vi "ExpStateLoadBridge.vi"(8 "Error In":errorcluster, 11 "Experiment State IN":T17={"error"={"status"=FALSE, "code"=0, "source"=""}, "Digitizer DAQmx Tasks"={"TaskArray"=[]}, "DAQ Settings"={"Channel Settings"=[], "Card Settings"=[]}, "Synchronization Settings"={"Synchronizer 0"="PXI1Slot2", "source terminal"="GlobalSoftwareTrigger", "Synchronizer 1"="PXI1Slot2"}, "DAQ Data"=[], "Next Shot#"="0", "System Message"="", "User Shot Notes"="", "Timing Settings"={"Timing Card Settings"=[], "Timing Channel Settings"=[[{"Delay (s)"=2.559999942779541, "Pulse width (s)"=0.009999999776482582, "Active"=TRUE, "Channel Name"="Fiber 8", "counter"="PXI1Slot8/ctr7", "FrontPanelTime"=2.559999942779541}]]}, "Timing Tasks"={"TaskArray"=[]}, "Tree"="0", "Time Card/Channels"=[2, 8], "DAQ Card/Channels"=[3, 8], "Program Version"="", "RIO Settings"={"Channel Settings"=[], "Card Settings"=[]}, "RIO References"={"Reference Array"=[]}, "RIO Data"={"RIO Deleaved Data"=[], "Raw Readout"=[]}, "RIO Card/Channels"=[3, 8], "DIO Channels"=0, "DIO Settings"={"DIO Channel Array"=[]}, "Global Settings"={"Initial Background Values"={"Reference Shot #"=0.0, "Background pressure [Torr]"=0.0, "Cryo temp [V]"=0.0, "Cryo temp [K]"=0.0, "Cryotemp Calibration File"=path ""}, "Gas Puffing"={"Gas A type"="N", "Gas B type"="N", "Gas C type"="N", "Gas A pressure [psi]"=0.0, "Gas B pressure [psi]"=0.0, "Gas C pressure [psi]"=0.0, "Innner Electrode"="", "Middle Electrode"="", "Outer Electrode"="", "Gas A bottle pressure [psi]"=0.0, "Gas B bottle pressure [psi]"=0.0, "Gas C bottle pressure [psi]"=0.0}, "PSU Voltages"={"Bias1 Voltage [V]"=0.0, "Bias2 Voltage [V]"=0.0, "PSU1 Voltage [V]"=0.0, "Puff-PSU1 CH1 Voltage [V]"=0.0, "Puff-PSU1 CH2 Voltage [V]"=0.0, "Puff-PSU1 CH3 Voltage [V]"=0.0, "PSU2 Voltage [V]"=0.0, "PSU3 Voltage [V]"=0.0}, "TEK 2024B - TEK - Details"={"CH1"="", "CH2"="", "CH3"="", "CH4"="", "CH1 Ground State"="Grounded", "CH2 Ground State"="Grounded", "CH3 Ground State"="Grounded", "CH4 Ground State"="Grounded"}, "TEK 2024B - TEK1 - Details"={"CH1"="", "CH2"="", "CH3"="", "CH4"="", "CH1 Ground State"="Grounded", "CH2 Ground State"="Grounded", "CH3 Ground State"="Grounded", "CH4 Ground State"="Grounded"}}, "Calibrations"={"CryoTemp"={"Comment"="", "X"=[], "Y"=[]}, "PSU2 Tach"={"Comment"="", "X"=[], "Y"=[]}, "PSU3 Tach"={"Comment"="", "X"=[], "Y"=[]}, "PSU2 RevTach"={"Comment"="", "X"=[], "Y"=[]}, "PSU3 RevTach"={"Comment"="", "X"=[], "Y"=[]}}, "Tach Tasks"={"PSU2 task"="", "PSU3 task"=""}, "PSU2 Panel Settings"={"PSU2 DIO channels"={"Charge relay DIO"="DAQ0/port0/line3", "Dump relay DIO"="DAQ0/port0/line4", "HV Arm DIO"="DAQ0/port0/line5", "HV On DIO"="DAQ0/port0/line6"}, "PSU2 Tachometer Controls"={"PSU2 Tach Calibration"=path "Z:/Data/Calibration/Tachometer", "PSU2 Charging Voltage [kV]"=0.0, "PSU2 Tach Counter"="DAQ0/port0/line3"}, "PSU2 Reverse Tachometer Controls"={"PSU2 RevTach Calibration"=path "Z:/Data/Calibration/Reverse Tachometer/PSU2_RevTachCalibration.csv", "PSU2 bank Voltage [kV]"=0.0, "PSU2 RevTach Counter"=""}}, "PSU3 Panel Settings"={"PSU3 DIO channels"={"Charge relay DIO"="DAQ0/port0/line5", "Dump relay DIO"="DAQ0/port0/line6", "HV Arm DIO"="", "HV On DIO"="DAQ0/port0/line6"}, "PSU3 Tachometer Controls"={"PSU3 Tach Calibration"=path "Z:/Data/Calibration/Reverse Tachometer/PSU3_RevTachCalibration.csv", "PSU3 Charging Voltage [kV]"=0.0, "PSU3 Tach Counter"=""}, "PSU3 Reverse Tachometer Controls"={"PSU3 RevTach Calibration"=path "Z:/Data/Calibration/Reverse Tachometer/PSU3_RevTachCalibration.csv", "PSU3 bank Voltage [kV]"=0.0, "PSU3 RevTach Counter"=""}}} {"Global Settings"."Initial Background Values"."Cryo temp [K]" format="%#_4g"; "RIO Settings"."Card Settings"."Digital High \nPass Filter k" items=["10"=21, "9"=19, "8"=17, "7"=15, "6"=13, "5"=11, "4"=9, "3"=7, "2"=5, "Off"=0]; "RIO Settings"."Card Settings"."Sample Rate" format="%#_3p"; "Timing Settings"."Timing Channel Settings"."FrontPanelTime" format="%.3p"; "Timing Settings"."Timing Channel Settings"."Pulse width (s)" format="%.3p"; "Timing Settings"."Timing Channel Settings"."Delay (s)" format="%.3p"; "DAQ Settings"."Card Settings"."Global Edge Type" items=["Rising"=10280, "Falling"=10171]; "DAQ Settings"."Card Settings"."Sample Rate" format="%#_3p"}) -> (0 "Load RIO Array":T7 {"Card Settings"."Digital High \nPass Filter k" items=["10"=21, "9"=19, "8"=17, "7"=15, "6"=13, "5"=11, "4"=9, "3"=7, "2"=5, "Off"=0]; "Card Settings"."Start Time" format="%#_3p"; "Card Settings"."End Time" format="%#_3p"; "Card Settings"."Rate" format="%#_3p"}, 1 "Load DAQ Array":T46(array[cluster]) {"Card Settings"."Start Time" format="%#_3p"; "Card Settings"."End Time" format="%#_3p"; "Card Settings"."Rate" format="%#_3p"}, 2 "Load Timing Array":T47[](array[typedef]) {"Timing Sequence"."Pulse Width [s]" format="%#.2p"; "Timing Sequence"."Dt" format="%.2p"; "Timing Sequence"."Time" format="%.2p"}, 3 "Experiment State OUT":T17={"error"={"status"=FALSE, "code"=0, "source"=""}, "Digitizer DAQmx Tasks"={"TaskArray"=[]}, "DAQ Settings"={"Channel Settings"=[], "Card Settings"=[]}, "Synchronization Settings"={"Synchronizer 0"="PXI1Slot2", "source terminal"="GlobalSoftwareTrigger", "Synchronizer 1"="PXI1Slot2"}, "DAQ Data"=[], "Next Shot#"="0", "System Message"="", "User Shot Notes"="", "Timing Settings"={"Timing Card Settings"=[], "Timing Channel Settings"=[[{"Delay (s)"=2.559999942779541, "Pulse width (s)"=0.009999999776482582, "Active"=TRUE, "Channel Name"="Fiber 8", "counter"="PXI1Slot8/ctr7", "FrontPanelTime"=2.559999942779541}]]}, "Timing Tasks"={"TaskArray"=[]}, "Tree"="0", "Time Card/Channels"=[2, 8], "DAQ Card/Channels"=[3, 8], "Program Version"="", "RIO Settings"={"Channel Settings"=[], "Card Settings"=[]}, "RIO References"={"Reference Array"=[]}, "RIO Data"={"RIO Deleaved Data"=[], "Raw Readout"=[]}, "RIO Card/Channels"=[3, 8], "DIO Channels"=0, "DIO Settings"={"DIO Channel Array"=[]}, "Global Settings"={"Initial Background Values"={"Reference Shot #"=0.0, "Background pressure [Torr]"=0.0, "Cryo temp [V]"=0.0, "Cryo temp [K]"=0.0, "Cryotemp Calibration File"=path ""}, "Gas Puffing"={"Gas A type"="N", "Gas B type"="N", "Gas C type"="N", "Gas A pressure [psi]"=0.0, "Gas B pressure [psi]"=0.0, "Gas C pressure [psi]"=0.0, "Innner Electrode"="", "Middle Electrode"="", "Outer Electrode"="", "Gas A bottle pressure [psi]"=0.0, "Gas B bottle pressure [psi]"=0.0, "Gas C bottle pressure [psi]"=0.0}, "PSU Voltages"={"Bias1 Voltage [V]"=0.0, "Bias2 Voltage [V]"=0.0, "PSU1 Voltage [V]"=0.0, "Puff-PSU1 CH1 Voltage [V]"=0.0, "Puff-PSU1 CH2 Voltage [V]"=0.0, "Puff-PSU1 CH3 Voltage [V]"=0.0, "PSU2 Voltage [V]"=0.0, "PSU3 Voltage [V]"=0.0}, "TEK 2024B - TEK - Details"={"CH1"="", "CH2"="", "CH3"="", "CH4"="", "CH1 Ground State"="Grounded", "CH2 Ground State"="Grounded", "CH3 Ground State"="Grounded", "CH4 Ground State"="Grounded"}, "TEK 2024B - TEK1 - Details"={"CH1"="", "CH2"="", "CH3"="", "CH4"="", "CH1 Ground State"="Grounded", "CH2 Ground State"="Grounded", "CH3 Ground State"="Grounded", "CH4 Ground State"="Grounded"}}, "Calibrations"={"CryoTemp"={"Comment"="", "X"=[], "Y"=[]}, "PSU2 Tach"={"Comment"="", "X"=[], "Y"=[]}, "PSU3 Tach"={"Comment"="", "X"=[], "Y"=[]}, "PSU2 RevTach"={"Comment"="", "X"=[], "Y"=[]}, "PSU3 RevTach"={"Comment"="", "X"=[], "Y"=[]}}, "Tach Tasks"={"PSU2 task"="", "PSU3 task"=""}, "PSU2 Panel Settings"={"PSU2 DIO channels"={"Charge relay DIO"="DAQ0/port0/line3", "Dump relay DIO"="DAQ0/port0/line4", "HV Arm DIO"="DAQ0/port0/line5", "HV On DIO"="DAQ0/port0/line6"}, "PSU2 Tachometer Controls"={"PSU2 Tach Calibration"=path "Z:/Data/Calibration/Tachometer", "PSU2 Charging Voltage [kV]"=0.0, "PSU2 Tach Counter"="DAQ0/port0/line3"}, "PSU2 Reverse Tachometer Controls"={"PSU2 RevTach Calibration"=path "Z:/Data/Calibration/Reverse Tachometer/PSU2_RevTachCalibration.csv", "PSU2 bank Voltage [kV]"=0.0, "PSU2 RevTach Counter"=""}}, "PSU3 Panel Settings"={"PSU3 DIO channels"={"Charge relay DIO"="DAQ0/port0/line5", "Dump relay DIO"="DAQ0/port0/line6", "HV Arm DIO"="", "HV On DIO"="DAQ0/port0/line6"}, "PSU3 Tachometer Controls"={"PSU3 Tach Calibration"=path "Z:/Data/Calibration/Reverse Tachometer/PSU3_RevTachCalibration.csv", "PSU3 Charging Voltage [kV]"=0.0, "PSU3 Tach Counter"=""}, "PSU3 Reverse Tachometer Controls"={"PSU3 RevTach Calibration"=path "Z:/Data/Calibration/Reverse Tachometer/PSU3_RevTachCalibration.csv", "PSU3 bank Voltage [kV]"=0.0, "PSU3 RevTach Counter"=""}}} {"Global Settings"."Initial Background Values"."Cryo temp [K]" format="%#_4g"; "RIO Settings"."Card Settings"."Digital High \nPass Filter k" items=["10"=21, "9"=19, "8"=17, "7"=15, "6"=13, "5"=11, "4"=9, "3"=7, "2"=5, "Off"=0]; "RIO Settings"."Card Settings"."Sample Rate" format="%#_3p"; "Timing Settings"."Timing Channel Settings"."FrontPanelTime" format="%.3p"; "Timing Settings"."Timing Channel Settings"."Pulse width (s)" format="%.3p"; "Timing Settings"."Timing Channel Settings"."Delay (s)" format="%.3p"; "DAQ Settings"."Card Settings"."Global Edge Type" items=["Rising"=10280, "Falling"=10171]; "DAQ Settings"."Card Settings"."Sample Rate" format="%#_3p"}, 4 "Load DIO Cluster":T14, 5 "Shot Notes":string, 6 "Global Settings":T2={"Initial Background Values"={"Reference Shot #"=0.0, "Background pressure [Torr]"=0.0, "Cryo temp [V]"=0.0, "Cryo temp [K]"=0.0, "Cryotemp Calibration File"=path ""}, "Gas Puffing"={"Gas A type"="N", "Gas B type"="N", "Gas C type"="N", "Gas A pressure [psi]"=0.0, "Gas B pressure [psi]"=0.0, "Gas C pressure [psi]"=0.0, "Innner Electrode"="", "Middle Electrode"="", "Outer Electrode"="", "Gas A bottle pressure [psi]"=0.0, "Gas B bottle pressure [psi]"=0.0, "Gas C bottle pressure [psi]"=0.0}, "PSU Voltages"={"Bias1 Voltage [V]"=0.0, "Bias2 Voltage [V]"=0.0, "PSU1 Voltage [V]"=0.0, "Puff-PSU1 CH1 Voltage [V]"=0.0, "Puff-PSU1 CH2 Voltage [V]"=0.0, "Puff-PSU1 CH3 Voltage [V]"=0.0, "PSU2 Voltage [V]"=0.0, "PSU3 Voltage [V]"=0.0}, "TEK 2024B - TEK - Details"={"CH1"="", "CH2"="", "CH3"="", "CH4"="", "CH1 Ground State"="Grounded", "CH2 Ground State"="Grounded", "CH3 Ground State"="Grounded", "CH4 Ground State"="Grounded"}, "TEK 2024B - TEK1 - Details"={"CH1"="", "CH2"="", "CH3"="", "CH4"="", "CH1 Ground State"="Grounded", "CH2 Ground State"="Grounded", "CH3 Ground State"="Grounded", "CH4 Ground State"="Grounded"}} {"Initial Background Values"."Cryo temp [K]" format="%#_4g"}, 9 "PSU2 Control Panel":T1={"HV Off State"=FALSE, "HV On State"=FALSE, "HV Arm"=FALSE, "HV On"=FALSE, "Charge relay DIO"="DAQ0/port0/line3", "Dump relay DIO"="DAQ0/port0/line4", "HV Arm DIO"="DAQ0/port0/line5", "HV On DIO"="DAQ0/port0/line6", "Bank Voltage [kV]"={0.0, 0.0}, "Vdemand Counter"="Timing1/ctr1", "RevTach Calibration"=path "Z:/Data/Calibration/Reverse Tachometer/PSU2_RevTachCalibration.csv", "Vdemand"=FALSE, "Vmeasure Counter"="Timing1/ctr2", "Tach Calibration"=path "Z:/Data/Calibration/Tachometer/PSU2_TachCalibration.csv", "Vmeasure"=FALSE, "Vdemand [kV]"=0.0, "Charge Relay"=FALSE, "Dump Relay"=FALSE} {"Bank Voltage [kV]" scale=0.01..10.0 scale format="%#_3g"}, 10 "PSU3 Control Panel":T1={"HV Off State"=FALSE, "HV On State"=FALSE, "HV Arm"=FALSE, "HV On"=FALSE, "Charge relay DIO"="DAQ0/port0/line3", "Dump relay DIO"="DAQ0/port0/line4", "HV Arm DIO"="DAQ0/port0/line5", "HV On DIO"="DAQ0/port0/line6", "Bank Voltage [kV]"={0.0, 0.0}, "Vdemand Counter"="Timing1/ctr1", "RevTach Calibration"=path "Z:/Data/Calibration/Reverse Tachometer/PSU2_RevTachCalibration.csv", "Vdemand"=FALSE, "Vmeasure Counter"="Timing1/ctr2", "Tach Calibration"=path "Z:/Data/Calibration/Tachometer/PSU2_TachCalibration.csv", "Vmeasure"=FALSE, "Vdemand [kV]"=0.0, "Charge Relay"=FALSE, "Dump Relay"=FALSE} {"Bank Voltage [kV]" scale=0.01..10.0 scale format="%#_3g"})   [LabVIEW 2015]
uses:
  Controls/TimingControl.ctl
  Controls/TimingControlChannel.ctl
  Controls/DAQ Card Channel Array.ctl
  Controls/DAQ Channel Settings.ctl
  Controls/DAQ Card Settings.ctl
  Controls/ExperimentStateCluster.ctl
  Controls/DigitizerSettingsChannelSettings.ctl
  Controls/DigitizerSettingsCardSettingsArray.ctl
  Controls/DigitizerSettingsCardSettings.ctl
  Controls/TimingSettings.ctl
  Controls/TimingCardSettings.ctl
  Controls/TimingChannelSettings.ctl
  Controls/RIOSettingsExperimentStateCluster.ctl
  Controls/RIOChannelSettingsArrayExperimentStateCluster.ctl
  Controls/RIOSettingsChannelSettings.ctl
  Controls/RIOSettingsCardSettingsArray.ctl
  Controls/RIOSettingsCardSettings.ctl
  <vilib>/userdefined/High Color/nirio_resource_hc.ctl
  Controls/DigitalHighPassFilter.ctl
  Controls/RIOData.ctl
  Controls/DIOChannel.ctl
  Controls/Global Settings/GlobalSettings.ctl
  Controls/Global Settings/InitialBackgroundValues.ctl
  Controls/Global Settings/GasPuffing.ctl
  Controls/Global Settings/PSUVoltages.ctl
  Controls/Global Settings/ScopeDetails.ctl
  Controls/Calibrations/Calibrations.ctl
  Controls/Calibrations/CryoTemoCalibration.ctl
  Controls/Calibrations/PSU2TachCalibration.ctl
  Controls/Calibrations/PSU3TachCalibration.ctl
  Controls/TachTasks.ctl
  Controls/PSU2PanelSettings.ctl
  Controls/PSU2DIOChannels.ctl
  Controls/PSU2TachometerControls.ctl
  Controls/PSU2ReverseTachometerControls.ctl
  Controls/PSU3PanelSettings.ctl
  Controls/PSU3DIOChannels.ctl
  Controls/PSU3TachometerControls.ctl
  Controls/PSU3ReverseTachometerControls.ctl
  Controls/DIOTypedef.ctl
  Controls/DIOChannelArray.ctl
  Controls/RIOCardArray.ctl
  Controls/RIOCardElement.ctl
  Controls/RIOCardChannelArray.ctl
  Controls/RIOChannelSettings.ctl
  Controls/RIOCardSettings.ctl
  Controls/PSUPanel-Arming.ctl
  Controls/DAQ Card-Channel Settings.ctl
panel:
  # "Channel                                                  Name                         Atten [dB]            Card Settings"
  # "Sampling Rate [1/s]"
  # "Start Time [s]"
  # "End Time [s]"
  # "On/Off      Channel                     Name"
  # "Sampling Rate [1/s]"
  # "Start Time [s]"
  # "End Time [s]"
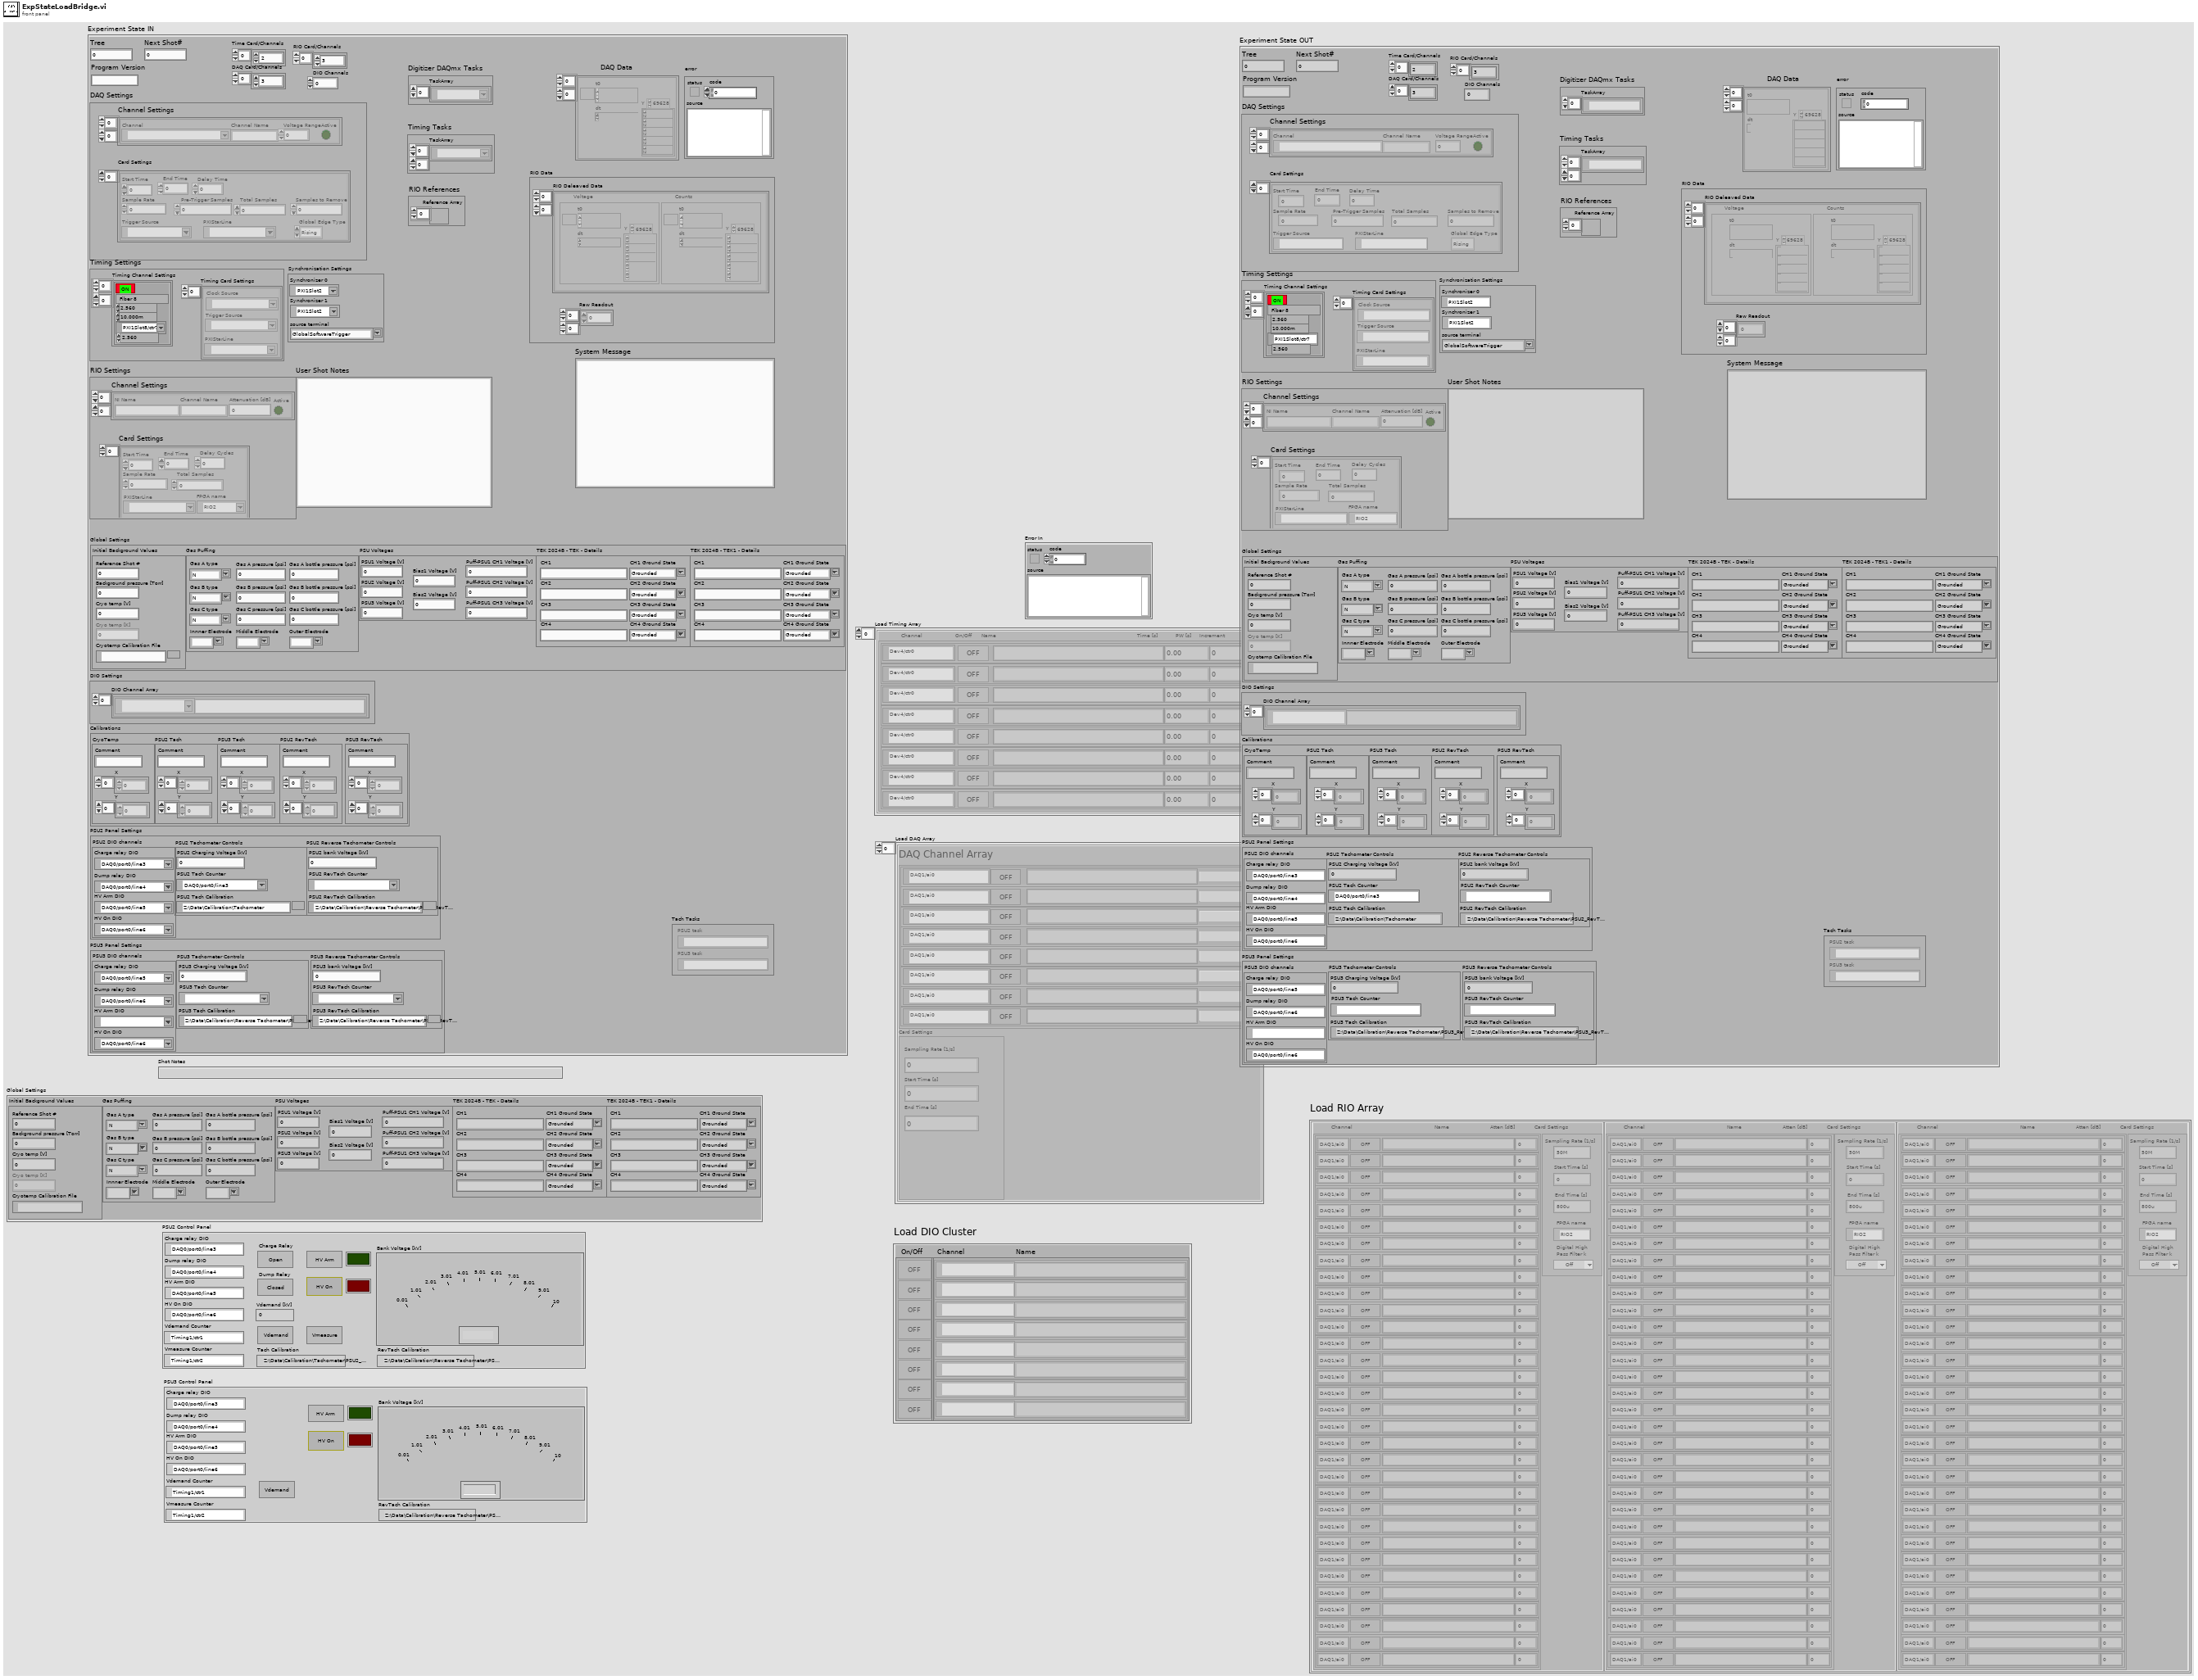
[diagram p1: front panel]
types:
  T1 = typedef "PSUPanel-Arming.ctl" = cluster{"HV Off State":bool, "HV On State":bool, "HV Arm":bool, "HV On":bool, "Charge relay DIO":tag, "Dump relay DIO":tag, "HV Arm DIO":tag, "HV On DIO":tag, "Bank Voltage [kV]":cluster{dbl, dbl}, "Vdemand Counter":tag, "RevTach Calibration":path, "Vdemand":bool, "Vmeasure Counter":tag, "Tach Calibration":path, "Vmeasure":bool, "Vdemand [kV]":dbl, "Charge Relay":bool, "Dump Relay":bool}
  T2 = typedef "GlobalSettings.ctl" = cluster{"Initial Background Values":T3, "Gas Puffing":T4, "PSU Voltages":T5, "TEK 2024B - TEK - Details":T6, "TEK 2024B - TEK1 - Details":T6}
  T3 = typedef "InitialBackgroundValues.ctl" = cluster{"Reference Shot #":dbl, "Background pressure [Torr]":dbl, "Cryo temp [V]":dbl, "Cryo temp [K]":dbl, "Cryotemp Calibration File":path}
  T4 = typedef "GasPuffing.ctl" = cluster{"Gas A type":string, "Gas B type":string, "Gas C type":string, "Gas A pressure [psi]":dbl, "Gas B pressure [psi]":dbl, "Gas C pressure [psi]":dbl, "Innner Electrode":string, "Middle Electrode":string, "Outer Electrode":string, "Gas A bottle pressure [psi]":dbl, "Gas B bottle pressure [psi]":dbl, "Gas C bottle pressure [psi]":dbl}
  T5 = typedef "PSUVoltages.ctl" = cluster{"Bias1 Voltage [V]":dbl, "Bias2 Voltage [V]":dbl, "PSU1 Voltage [V]":dbl, "Puff-PSU1 CH1 Voltage [V]":dbl, "Puff-PSU1 CH2 Voltage [V]":dbl, "Puff-PSU1 CH3 Voltage [V]":dbl, "PSU2 Voltage [V]":dbl, "PSU3 Voltage [V]":dbl}
  T6 = typedef "ScopeDetails.ctl" = cluster{"CH1":string, "CH2":string, "CH3":string, "CH4":string, "CH1 Ground State":string, "CH2 Ground State":string, "CH3 Ground State":string, "CH4 Ground State":string}
  T7 = typedef "RIOCardArray.ctl" = T8[][]
  T8 = typedef "RIOCardElement.ctl" = cluster{"RIO Channel Array":T9, "Card Settings":T11}
  T9 = typedef "RIOCardChannelArray.ctl" = T10[]
  T10 = typedef "RIOChannelSettings.ctl" = cluster{"Active":bool, "Channel Name":string, "NI Name":string, "Attenutaion [dB]":i32}
  T11 = typedef "RIOCardSettings.ctl" = cluster{"Rate":dbl, "End Time":dbl, "Start Time":dbl, "FPGA name":T12, "Digital High \nPass Filter k":T13}
  T12 = typedef "nirio_resource_hc.ctl" = tag
  T13 = typedef "DigitalHighPassFilter.ctl" = u16
  T14 = typedef "DIOTypedef.ctl" = cluster{"DIO Booleans":bool[], "DIO Channel Array":T15}
  T15 = typedef "DIOChannelArray.ctl" = T16[]
  T16 = typedef "DIOChannel.ctl" = cluster{"Channel Name":string, "NI Name":tag}
  T17 = typedef "ExperimentStateCluster.ctl" = cluster{"error":errorcluster, "Digitizer DAQmx Tasks":cluster{"TaskArray":refnum<k21>[]}, "DAQ Settings":cluster{"Channel Settings":T18[][], "Card Settings":T19}, "Synchronization Settings":cluster{"Synchronizer 0":refnum<k15>, "source terminal":string, "Synchronizer 1":refnum<k15>}, "DAQ Data":waveform(dbl)[][], "Next Shot#":string, "System Message":string, "User Shot Notes":string, "Timing Settings":T21, "Timing Tasks":cluster{"TaskArray":refnum<k21>[][]}, "Tree":string, "Time Card/Channels":i32[], "DAQ Card/Channels":i32[], "Program Version":string, "RIO Settings":T24, "RIO References":cluster{"Reference Array":refnum<k20>[]}, "RIO Data":T29, "RIO Card/Channels":i32[], "DIO Channels":i32, "DIO Settings":cluster{"DIO Channel Array":T16[]}, "Global Settings":T2, "Calibrations":T30, "Tach Tasks":T34, "PSU2 Panel Settings":T35, "PSU3 Panel Settings":T39}
  T18 = typedef "DigitizerSettingsChannelSettings.ctl" = cluster{"Channel":tag, "Channel Name":string, "Voltage Range":dbl, "Active":bool}
  T19 = typedef "DigitizerSettingsCardSettingsArray.ctl" = T20[]
  T20 = typedef "DigitizerSettingsCardSettings.ctl" = cluster{"Start Time":dbl, "End Time":dbl, "Sample Rate":dbl, " Pre-Trigger Samples":u32, "Total Samples":i32, "Samples to Remove":u32, "Trigger Source":tag, "Global Edge Type":i32, "PXIStarLine":tag, "Delay Time":dbl}
  T21 = typedef "TimingSettings.ctl" = cluster{"Timing Card Settings":T22[], "Timing Channel Settings":T23[][]}
  T22 = typedef "TimingCardSettings.ctl" = cluster{"Trigger Source":tag, "Clock Source":tag, "PXIStarLine":tag}
  T23 = typedef "TimingChannelSettings.ctl" = cluster{"Delay (s)":dbl, "Pulse width (s)":dbl, "Active":bool, "Channel Name":string, "counter":tag, "FrontPanelTime":dbl}
  T24 = typedef "RIOSettingsExperimentStateCluster.ctl" = cluster{"Channel Settings":T25, "Card Settings":T27}
  T25 = typedef "RIOChannelSettingsArrayExperimentStateCluster.ctl" = T26[][]
  T26 = typedef "RIOSettingsChannelSettings.ctl" = cluster{"Channel Name":string, "Active":bool, "NI Name":string, "Attenuation [dB]":i32}
  T27 = typedef "RIOSettingsCardSettingsArray.ctl" = T28[]
  T28 = typedef "RIOSettingsCardSettings.ctl" = cluster{"Start Time":dbl, "End Time":dbl, "Sample Rate":dbl, "Total Samples":u64, "PXIStarLine":tag, "Delay Cycles":u64, "FPGA name":T12, "Digital High \nPass Filter k":T13}
  T29 = typedef "RIOData.ctl" = cluster{"RIO Deleaved Data":cluster{"Voltage":waveform(dbl), "Counts":waveform(i16)}[][], "Raw Readout":u64[][]}
  T30 = typedef "Calibrations.ctl" = cluster{"CryoTemp":T31, "PSU2 Tach":T32, "PSU3 Tach":T33, "PSU2 RevTach":T32, "PSU3 RevTach":T33}
  T31 = typedef "CryoTemoCalibration.ctl" = cluster{"Comment":string, "X":dbl[], "Y":dbl[]}
  T32 = typedef "PSU2TachCalibration.ctl" = cluster{"Comment":string, "X":dbl[], "Y":dbl[]}
  T33 = typedef "PSU3TachCalibration.ctl" = cluster{"Comment":string, "X":dbl[], "Y":dbl[]}
  T34 = typedef "TachTasks.ctl" = cluster{"PSU2 task":refnum<k21>, "PSU3 task":refnum<k21>}
  T35 = typedef "PSU2PanelSettings.ctl" = cluster{"PSU2 DIO channels":T36, "PSU2 Tachometer Controls":T37, "PSU2 Reverse Tachometer Controls":T38}
  T36 = typedef "PSU2DIOChannels.ctl" = cluster{"Charge relay DIO":tag, "Dump relay DIO":tag, "HV Arm DIO":tag, "HV On DIO":tag}
  T37 = typedef "PSU2TachometerControls.ctl" = cluster{"PSU2 Tach Calibration":path, "PSU2 Charging Voltage [kV]":dbl, "PSU2 Tach Counter":tag}
  T38 = typedef "PSU2ReverseTachometerControls.ctl" = cluster{"PSU2 RevTach Calibration":path, "PSU2 bank Voltage [kV]":dbl, "PSU2 RevTach Counter":tag}
  T39 = typedef "PSU3PanelSettings.ctl" = cluster{"PSU3 DIO channels":T40, "PSU3 Tachometer Controls":T41, "PSU3 Reverse Tachometer Controls":T42}
  T40 = typedef "PSU3DIOChannels.ctl" = cluster{"Charge relay DIO":tag, "Dump relay DIO":tag, "HV Arm DIO":tag, "HV On DIO":tag}
  T41 = typedef "PSU3TachometerControls.ctl" = cluster{"PSU3 Tach Calibration":path, "PSU3 Charging Voltage [kV]":dbl, "PSU3 Tach Counter":tag}
  T42 = typedef "PSU3ReverseTachometerControls.ctl" = cluster{"PSU3 RevTach Calibration":path, "PSU3 bank Voltage [kV]":dbl, "PSU3 RevTach Counter":tag}
  T43 = typedef "DAQ Card Channel Array.ctl" = T44[]
  T44 = typedef "DAQ Channel Settings.ctl" = cluster{"Active":bool, "Channel Name":string, "Channel":tag, "Voltage Range":string}
  T45 = typedef "DAQ Card Settings.ctl" = cluster{"Rate":dbl, "End Time":dbl, "Start Time":dbl}
  T46 = cluster{"DAQ Channel Array":T43, "Card Settings":T45}[]
  T47 = typedef "TimingControl.ctl" = cluster{"Timing Sequence":T48[]}
  T48 = typedef "TimingControlChannel.ctl" = cluster{"Active":bool, "counter":tag, "Channel Name":string, "Time":dbl, "Increment":string, "Dt":dbl, "Pulse Width [s]":dbl}
  T49 = typedef "DAQ Card-Channel Settings.ctl" = cluster{"DAQ Channel Array":T43, "Card Settings":T45}
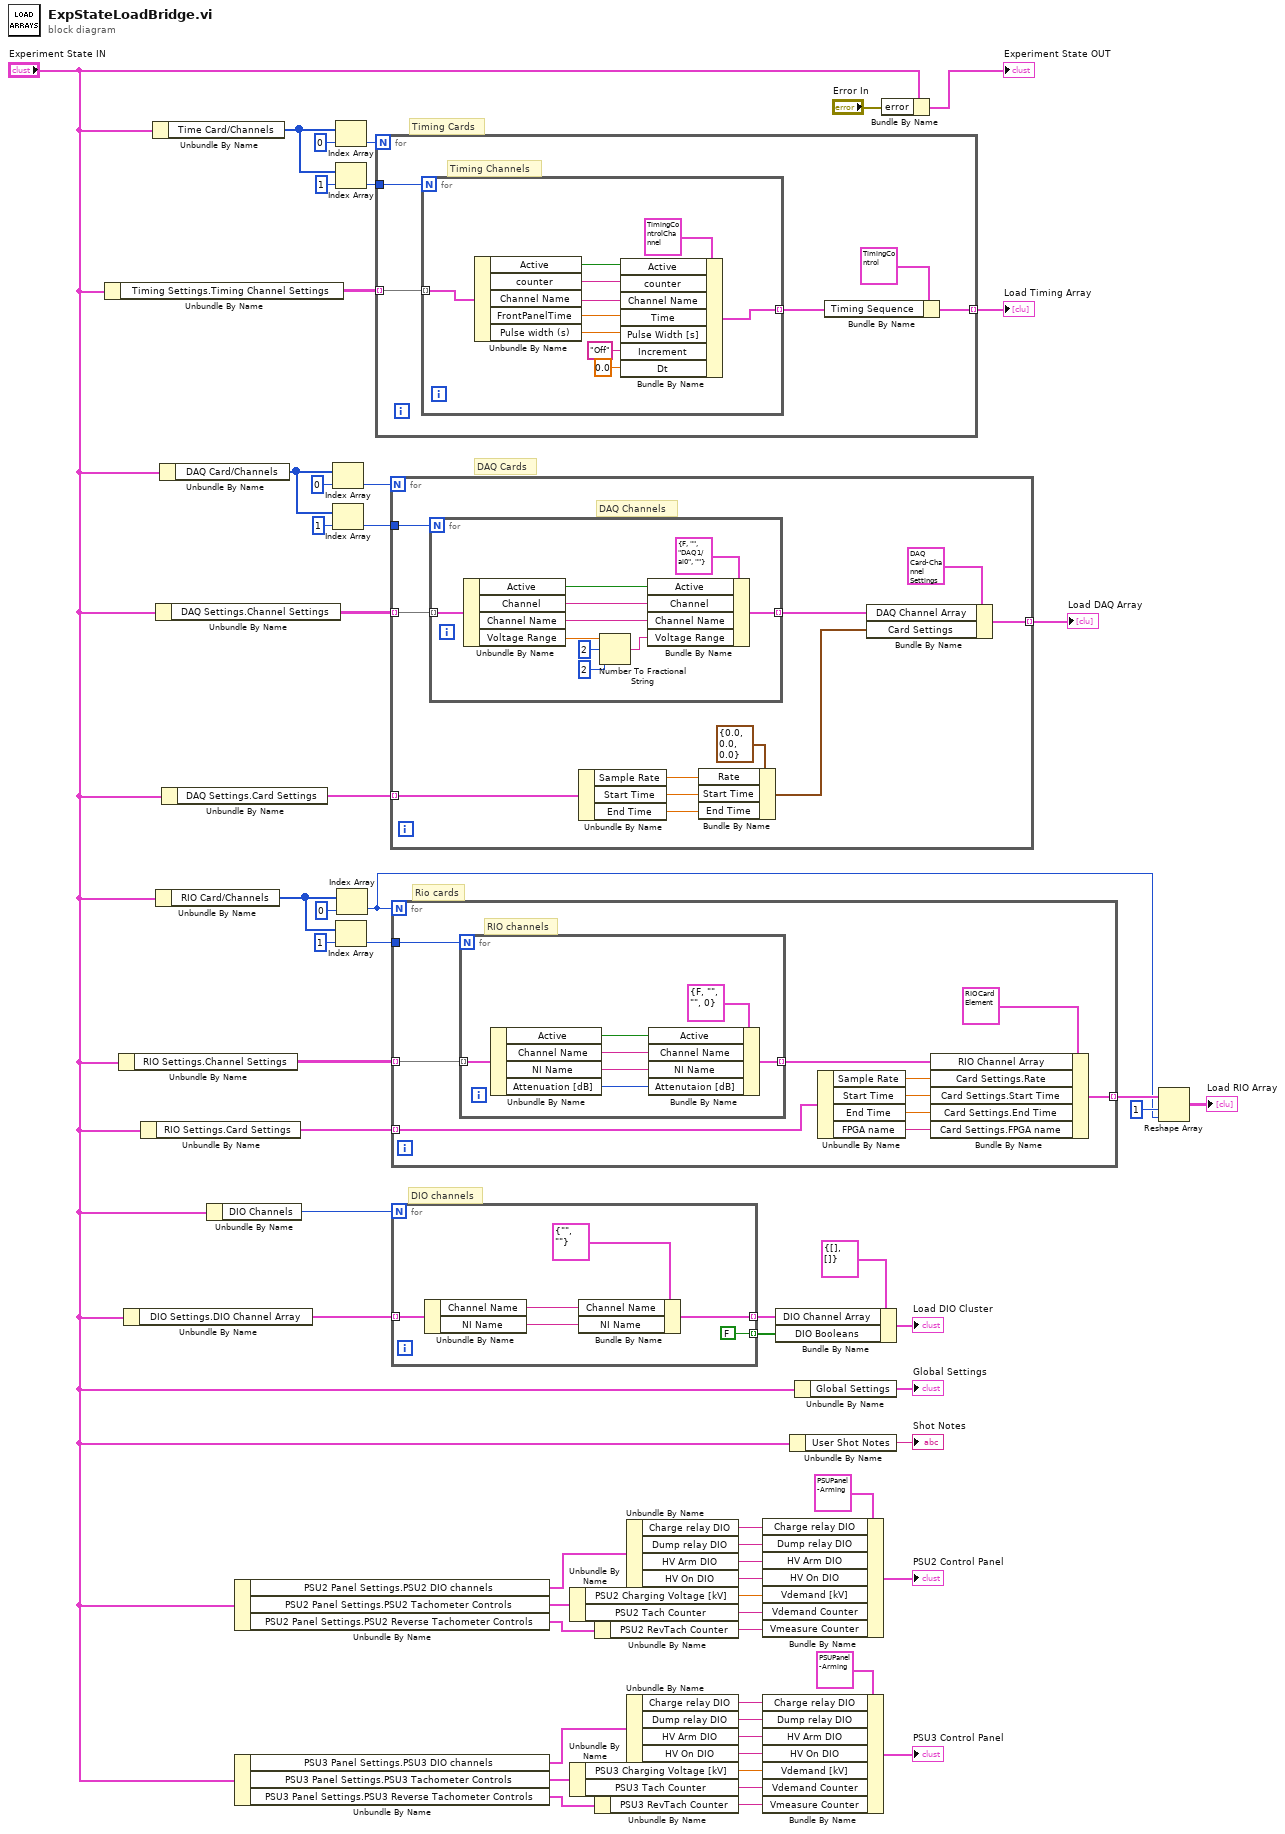
[diagram p0: block diagram]
diagram:
  # "DIO channels"
  # "Rio cards"
  # "DAQ Cards"
  # "Timing Cards"
  n1 = Unbundle By Name("Experiment State IN") -> ("Timing Settings.Timing Channel Settings"=w53:T23[][])
  n2 = Unbundle By Name("Experiment State IN") -> ("RIO Settings.Channel Settings"=w39:T25)
  n3 = Unbundle By Name("Experiment State IN") -> ("DIO Settings.DIO Channel Array"=w36:T16[])
  n4 = Unbundle By Name("Experiment State IN") -> ("RIO Settings.Card Settings"=w38:T27)
  n5 = Unbundle By Name("Experiment State IN") -> ("Time Card/Channels"=w55:i32[])
  n6 = Unbundle By Name("Experiment State IN") -> ("DAQ Settings.Channel Settings"=w47:T18[][])
  n7 = Unbundle By Name("Experiment State IN") -> ("RIO Card/Channels"=w40:i32[])
  n8 = Unbundle By Name("Experiment State IN") -> ("DAQ Card/Channels"=w50:i32[])
  n9 = Unbundle By Name("Experiment State IN") -> ("DAQ Settings.Card Settings"=w46:T19)
  n10 = Unbundle By Name("Experiment State IN") -> ("DIO Channels"=w37:i32)
  n11 = Unbundle By Name("Experiment State IN") -> ("PSU2 Panel Settings.PSU2 DIO channels"=w21:T36, "PSU2 Panel Settings.PSU2 Tachometer Controls"=w20:T37, "PSU2 Panel Settings.PSU2 Reverse Tachometer Controls"=w19:T38)
  n12 = Unbundle By Name("Experiment State IN") -> ("PSU3 Panel Settings.PSU3 DIO channels"=w9:T40, "PSU3 Panel Settings.PSU3 Tachometer Controls"=w8:T41, "PSU3 Panel Settings.PSU3 Reverse Tachometer Controls"=w7:T42)
  n13 = Index Array(array=w50, index=0) -> (element=w49:i32)
  n14 = Index Array(array=w50, index=1) -> (element=w48:i32)
  n15 = Index Array(array=w55, index=0) -> (element=w58:i32)
  n16 = Index Array(array=w55, index=1) -> (element=w54:i32)
  n17 = Index Array(array=w40, index=1) -> (element=w41:i32)
  n18 = Index Array(array=w40, index=0) -> (element=w28:i32)
  n19 = for {
    N: w58 -> [_]
    tunnel: [w65] -> w60 mode=indexing
    tunnel: w54 -> [w62]
    tunnel: w53 -> [w61] mode=indexing
    # "Timing Channels"
    n20 = for {
      N: w62 -> [_]
      tunnel: [w75] -> w63 mode=indexing
      tunnel: w61 -> [w74] mode=indexing
      n21 = Unbundle By Name(w74) -> ("Active"=w69:bool, "counter"=w72:tag, "Channel Name"=w71:string, "FrontPanelTime"=w70:dbl, "Pulse width (s)"=w68:dbl)
      n22 = Bundle By Name(cluster=T48 {"Active"=FALSE, "counter"="PXI1Slot9/ctr7", "Channel Name"="", "Time"=0.0, "Increment"="Off", "Dt"=0.0, "Pulse Width [s]"=0.0} ("Counters"), "Active"=w69, "counter"=w72, "Channel Name"=w71, "Time"=w70, "Pulse Width [s]"=w68, "Increment"="Off", "Dt"=0.0) -> (w75:T48)
    }
    n23 = Bundle By Name(cluster=T47 {"Timing Sequence"=[{"Active"=FALSE, "counter"="PXI1Slot9/ctr7", "Channel Name"="", "Time"=0.0, "Increment"="Off", "Dt"=0.0, "Pulse Width [s]"=0.0}, {"Active"=FALSE, "counter"="Dev4/ctr0", "Channel Name"="", "Time"=0.0, "Increment"="Off", "Dt"=0.0, "Pulse Width [s]"=0.0}, {"Active"=FALSE, "counter"="Dev4/ctr0", "Channel Name"="", "Time"=0.0, "Increment"="Off", "Dt"=0.0, "Pulse Width [s]"=0.0}, {"Active"=FALSE, "counter"="Dev4/ctr0", "Channel Name"="", "Time"=0.0, "Increment"="Off", "Dt"=0.0, "Pulse Width [s]"=0.0}, {"Active"=FALSE, "counter"="Dev4/ctr0", "Channel Name"="", "Time"=0.0, "Increment"="Off", "Dt"=0.0, "Pulse Width [s]"=0.0}, {"Active"=FALSE, "counter"="Dev4/ctr0", "Channel Name"="", "Time"=0.0, "Increment"="Off", "Dt"=0.0, "Pulse Width [s]"=0.0}, {"Active"=FALSE, "counter"="Dev4/ctr0", "Channel Name"="", "Time"=0.0, "Increment"="Off", "Dt"=0.0, "Pulse Width [s]"=0.0}, {"Active"=FALSE, "counter"="Dev4/ctr0", "Channel Name"="", "Time"=0.0, "Increment"="Off", "Dt"=0.0, "Pulse Width [s]"=0.0}]} ("Cluster"), "Timing Sequence"=w63) -> (w65:T47)
  }
  "Load Timing Array" <- w60
  n24 = for {
    N: w49 -> [_]
    tunnel: [w86] -> w59 mode=indexing
    tunnel: w48 -> [w83]
    tunnel: w47 -> [w82] mode=indexing
    tunnel: w46 -> [w80] mode=indexing
    # "DAQ Channels"
    n25 = for {
      N: w83 -> [_]
      tunnel: [w96] -> w84 mode=indexing
      tunnel: w82 -> [w95] mode=indexing
      n26 = Unbundle By Name(w95) -> ("Active"=w87:bool, "Channel"=w92:tag, "Channel Name"=w93:string, "Voltage Range"=w90:dbl)
      n27 = Number To Fractional String(number=w90, width (-)=i16 2, precision (6)=i16 2) -> (F-format string=w91:string)  [unwired: 1 in]
      n28 = Bundle By Name(cluster=T44 {"Active"=FALSE, "Channel Name"="", "Channel"="DAQ1/ai0", "Voltage Range"=""} ("Counters"), "Active"=w87, "Channel"=w92, "Channel Name"=w93, "Voltage Range"=w91) -> (w96:T44)
    }
    n29 = Unbundle By Name(w80) -> ("Sample Rate"=w76:dbl, "Start Time"=w77:dbl, "End Time"=w78:dbl)
    n30 = Bundle By Name(cluster=T45 {"Rate"=0.0, "End Time"=0.0, "Start Time"=0.0} ("Card Settings"), "Rate"=w76, "Start Time"=w77, "End Time"=w78) -> (w81:T45)
    n31 = Bundle By Name(cluster=T49 {"DAQ Channel Array"=[{"Active"=FALSE, "Channel Name"="", "Channel"="DAQ1/ai0", "Voltage Range"=""}, {"Active"=FALSE, "Channel Name"="", "Channel"="DAQ1/ai0", "Voltage Range"=""}, {"Active"=FALSE, "Channel Name"="", "Channel"="DAQ1/ai0", "Voltage Range"=""}, {"Active"=FALSE, "Channel Name"="", "Channel"="DAQ1/ai0", "Voltage Range"=""}, {"Active"=FALSE, "Channel Name"="", "Channel"="DAQ1/ai0", "Voltage Range"=""}, {"Active"=FALSE, "Channel Name"="", "Channel"="DAQ1/ai0", "Voltage Range"=""}, {"Active"=FALSE, "Channel Name"="", "Channel"="DAQ1/ai0", "Voltage Range"=""}, {"Active"=FALSE, "Channel Name"="", "Channel"="DAQ1/ai0", "Voltage Range"=""}], "Card Settings"={"Rate"=100.0, "End Time"=0.0, "Start Time"=0.0}} ("Cluster"), "DAQ Channel Array"=w84, "Card Settings"=w81) -> (w86:T49)
  }
  "Load DAQ Array" <- w59
  n32 = for {
    N: w28 -> [_]
    tunnel: w41 -> [w106]
    tunnel: [w103] -> w34 mode=indexing
    tunnel: w39 -> [w98] mode=indexing
    tunnel: w38 -> [w97] mode=indexing
    # "RIO channels"
    n33 = for {
      N: w106 -> [_]
      tunnel: [w113] -> w104 mode=indexing
      tunnel: w98 -> [w112] mode=indexing
      n34 = Unbundle By Name(w112) -> ("Active"=w110:bool, "Channel Name"=w109:string, "NI Name"=w108:string, "Attenuation [dB]"=w107:i32)
      n35 = Bundle By Name(cluster=T10 {"Active"=FALSE, "Channel Name"="", "NI Name"="", "Attenutaion [dB]"=0} ("Counters"), "Active"=w110, "Channel Name"=w109, "NI Name"=w108, "Attenutaion [dB]"=w107) -> (w113:T10)
    }
    n36 = Unbundle By Name(w97) -> ("Sample Rate"=w102:dbl, "Start Time"=w101:dbl, "End Time"=w100:dbl, "FPGA name"=w99:T12)
    n37 = Bundle By Name(cluster=T8 {"RIO Channel Array"=[], "Card Settings"={"Rate"=100.0, "End Time"=0.0, "Start Time"=0.0, "FPGA name"="RIO2", "Digital High \nPass Filter k"=0}} ("Cluster"), "RIO Channel Array"=w104, "Card Settings.Rate"=w102, "Card Settings.Start Time"=w101, "Card Settings.End Time"=w100, "Card Settings.FPGA name"=w99) -> (w103:T8)
  }
  n38 = for {
    N: w37 -> [_]
    tunnel: [w119] -> w30 mode=indexing
    tunnel: w36 -> [w118] mode=indexing
    tunnel: [FALSE ("Active")] -> w29 mode=indexing
    n39 = Unbundle By Name(w118) -> ("Channel Name"=w116:string, "NI Name"=w115:tag)
    n40 = Bundle By Name(cluster=T16 {"Channel Name"="", "NI Name"=""} ("DIO Channels"), "Channel Name"=w116, "NI Name"=w115) -> (w119:T16)
  }
  n41 = Unbundle By Name(w20) -> ("PSU2 Charging Voltage [kV]"=w14:dbl, "PSU2 Tach Counter"=w13:tag)
  n42 = Unbundle By Name(w8) -> ("PSU3 Charging Voltage [kV]"=w3:dbl, "PSU3 Tach Counter"=w2:tag)
  n43 = Unbundle By Name(w19) -> ("PSU2 RevTach Counter"=w12:tag)
  n44 = Unbundle By Name(w7) -> ("PSU3 RevTach Counter"=w1:tag)
  n45 = Unbundle By Name(w21) -> ("Charge relay DIO"=w18:tag, "Dump relay DIO"=w17:tag, "HV Arm DIO"=w16:tag, "HV On DIO"=w15:tag)
  n46 = Unbundle By Name(w9) -> ("Charge relay DIO"=w11:tag, "Dump relay DIO"=w6:tag, "HV Arm DIO"=w5:tag, "HV On DIO"=w4:tag)
  n47 = Bundle By Name(cluster=T1 {"HV Off State"=FALSE, "HV On State"=FALSE, "HV Arm"=FALSE, "HV On"=FALSE, "Charge relay DIO"="DAQ0/port0/line3", "Dump relay DIO"="DAQ0/port0/line4", "HV Arm DIO"="DAQ0/port0/line5", "HV On DIO"="DAQ0/port0/line6", "Bank Voltage [kV]"={0.0, 0.0}, "Vdemand Counter"="Timing1/ctr1", "RevTach Calibration"=path "Z:/Data/Calibration/Reverse Tachometer/PSU2_RevTachCalibration.csv", "Vdemand"=FALSE, "Vmeasure Counter"="Timing1/ctr2", "Tach Calibration"=path "Z:/Data/Calibration/Tachometer/PSU2_TachCalibration.csv", "Vmeasure"=FALSE, "Vdemand [kV]"=0.0, "Charge Relay"=FALSE, "Dump Relay"=FALSE} ("PSU Panel - Arming"), "Charge relay DIO"=w18, "Dump relay DIO"=w17, "HV Arm DIO"=w16, "HV On DIO"=w15, "Vdemand [kV]"=w14, "Vdemand Counter"=w13, "Vmeasure Counter"=w12) -> (→"PSU2 Control Panel":T1)
  n48 = Bundle By Name(cluster=T1 {"HV Off State"=FALSE, "HV On State"=FALSE, "HV Arm"=FALSE, "HV On"=FALSE, "Charge relay DIO"="DAQ0/port0/line3", "Dump relay DIO"="DAQ0/port0/line4", "HV Arm DIO"="DAQ0/port0/line5", "HV On DIO"="DAQ0/port0/line6", "Bank Voltage [kV]"={0.0, 0.0}, "Vdemand Counter"="Timing1/ctr1", "RevTach Calibration"=path "Z:/Data/Calibration/Reverse Tachometer/PSU2_RevTachCalibration.csv", "Vdemand"=FALSE, "Vmeasure Counter"="Timing1/ctr2", "Tach Calibration"=path "Z:/Data/Calibration/Tachometer/PSU2_TachCalibration.csv", "Vmeasure"=FALSE, "Vdemand [kV]"=0.0, "Charge Relay"=FALSE, "Dump Relay"=FALSE} ("PSU Panel - Arming"), "Charge relay DIO"=w11, "Dump relay DIO"=w6, "HV Arm DIO"=w5, "HV On DIO"=w4, "Vdemand [kV]"=w3, "Vdemand Counter"=w2, "Vmeasure Counter"=w1) -> (→"PSU3 Control Panel":T1)
  n49 = Bundle By Name(cluster=T14 {"DIO Booleans"=[], "DIO Channel Array"=[]} ("DIO Cluster"), "DIO Channel Array"=w30, "DIO Booleans"=w29) -> (→"Load DIO Cluster":T14)
  n50 = Unbundle By Name("Experiment State IN") -> ("User Shot Notes"=→"Shot Notes":string)
  n51 = Unbundle By Name("Experiment State IN") -> ("Global Settings"=→"Global Settings":T2)
  n52 = Bundle By Name(cluster="Experiment State IN", "error"="Error In") -> (→"Experiment State OUT":T17)
  n53 = Reshape Array(w34, 1 ("dimension size"), w28) -> (→"Load RIO Array":T8[][])
